vi "Read (Multiple Waveforms).vi"(8 "error in (no error)":errorcluster, 9 "Timeout (10000 ms)":u32=10000, 10 "Channels":u16[](array[ring]) items=["Channel 1", "Channel 2", "Channel 3", "Channel 4", "Math", "Reference A", "Reference B", "Reference C", "Reference D", "FFT"], 11 "VISA resource name":refnum<visa-resource-name>) -> (0 "error out":errorcluster, 2 "Waveform Data":waveform(dbl)[](graph), 3 "VISA resource name out":refnum<visa-resource-name>)   [LabVIEW 2014, in "Tektronix TDS 200 1000 2000 Series.lvlib"]
doc: "Initiates an acquisition on all channels that you enabled with the <B>Configure Channel</B> VI. The VI waits for the acquisition to complete and returns the waveform for the <B>Source Channels</B> you specified. If the oscilloscope did not complete the acquisition within the time period you specify with the Timeout parameter, the VI returns a timeout error. A common cause for a timeout error is the acquisition was not triggered. For example, the trigger level is out of range of the waveform. \n\n<b>Note(s):</b>\nIf your instrument does not support auto compensation for probe attenuation, you may need to adjust the scaling of the Waveform Data accordingly. This is handled automatically in the <B>Configure Channel</B> VI or can be done manually by multiplying the Waveform Data by the probe attenuation."
uses:
  <instrlib>/Tektronix TDS 200 1000 2000 Series/Tektronix TDS 200 1000 2000 Series.lvlib
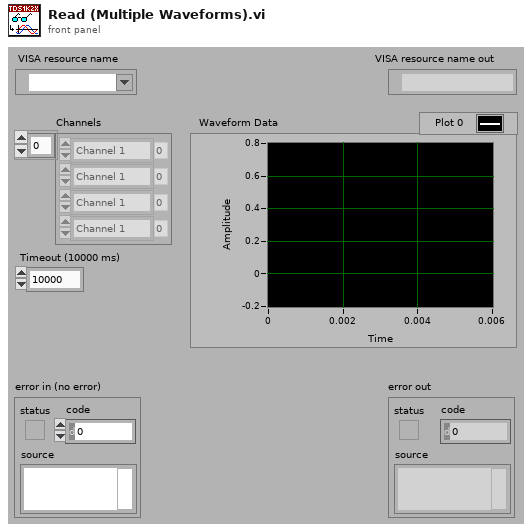
[diagram p1: front panel]
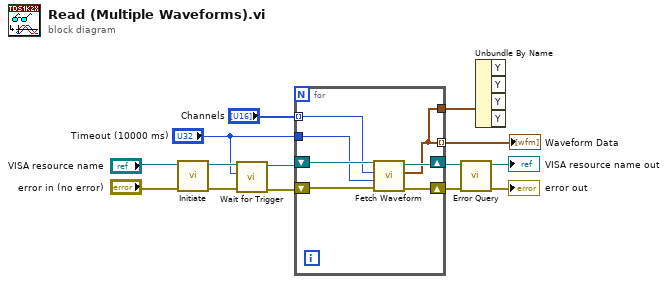
[diagram p0: block diagram]
diagram:
  n1 = call <instrlib>:"Initiate.vi"("error in (no error)"="error in (no error)", "VISA resource name"="VISA resource name") -> ("error out"=w3:errorcluster, "VISA resource name out"=w6:refnum<visa-resource-name>)  [unwired: 8 out]
  n2 = call <instrlib>:"Wait for Trigger.vi"("error in (no error)"=w3, "Timeout (10000 ms)"="Timeout (10000 ms)", "VISA resource name"=w6) -> ("error out"=w4:errorcluster, "VISA resource name out"=w5:refnum<visa-resource-name>)  [unwired: 7 out]
  n3 = for {
    shift-right: [w20] -> w11
    shift-left: w4 -> [w18]
    tunnel: "Channels" -> [w16] mode=indexing
    tunnel: [w15] -> w7 mode=indexing
    tunnel: "Timeout (10000 ms)" -> [w17]
    shift-right: [w21] -> w12
    shift-left: w5 -> [w19]
    tunnel: [w15] -> w1
    n4 = call <instrlib>:"Fetch Waveform.vi"("error in (no error)"=w18, "Timeout (10000 ms)"=w17, "Source (0: Channel 1)"=w16, "VISA resource name"=w19) -> ("error out"=w20:errorcluster, "Waveform Data"=w15:waveform(dbl), "VISA resource name out"=w21:refnum<visa-resource-name>)  [unwired: 2 in, 3 out]
  }
  "Waveform Data" <- w7
  n5 = call <instrlib>:"Error Query.vi"("error in (no error)"=w11, "VISA resource name"=w12) -> ("error out"=→"error out":errorcluster, "VISA resource name out"=→"VISA resource name out":refnum<visa-resource-name>)  [unwired: 8 out]
  n6 = Unbundle By Name(w1) -> ()  [unwired: 4 out]
